vi "Signal_Gen.vi"(8 "Iteraciones":i64, 9 "entrada":i64, 10 "Entrada":dbl[](array[numeric]), 11 "F":u32) -> (0 "salida_shift_reg":i64, 3 "Salida":u8)   [LabVIEW 2025]
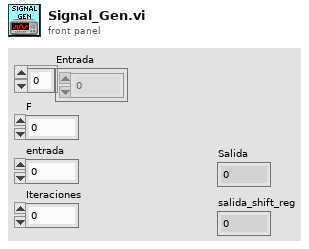
[diagram p1: front panel]
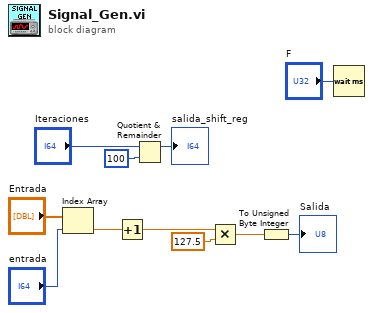
[diagram p0: block diagram]
diagram:
  n1 = Index Array(array="Entrada", index="entrada") -> (element=w8:dbl)
  n2 = Increment(x=w8) -> (x+1=w11:dbl)
  n3 = Quotient & Remainder(x="Iteraciones", y=100) -> (x-y*floor(x/y)=→"salida_shift_reg":i64)  [unwired: 1 out]
  n4 = Multiply(x=w11, y=127.5) -> (x*y=w7:dbl)
  n5 = To Unsigned Byte Integer(number=w7) -> (unsigned 8bit integer=→"Salida":u8)
  n6 = Wait (ms)(milliseconds to wait="F") -> ()  [unwired: 1 out]
